vi "Compile.vi"(6 "Python version":string="3.9", 7 "Console":refnum<vi>, 8 "error in":errorcluster, 9 "Code":string="   void setup() {\n    pinMode(LED_BUILTIN, OUTPUT);\n}\n\n   void loop() {\n     digitalWrite(LED_BUILTIN, HIGH);\n     delay(1000);\n     digitalWrite(LED_BUILTIN, LOW);\n     delay(1000);\n}\n", 11 "Arduino in":T1) -> (0 "error out":errorcluster, 1 "standard error":string, 2 "Reply":string, 3 "Arduino out":T1)   [LabVIEW 2022 SP3]
uses:
  ArduinoCtrl.ctl
panel:
  out "resulting string":string
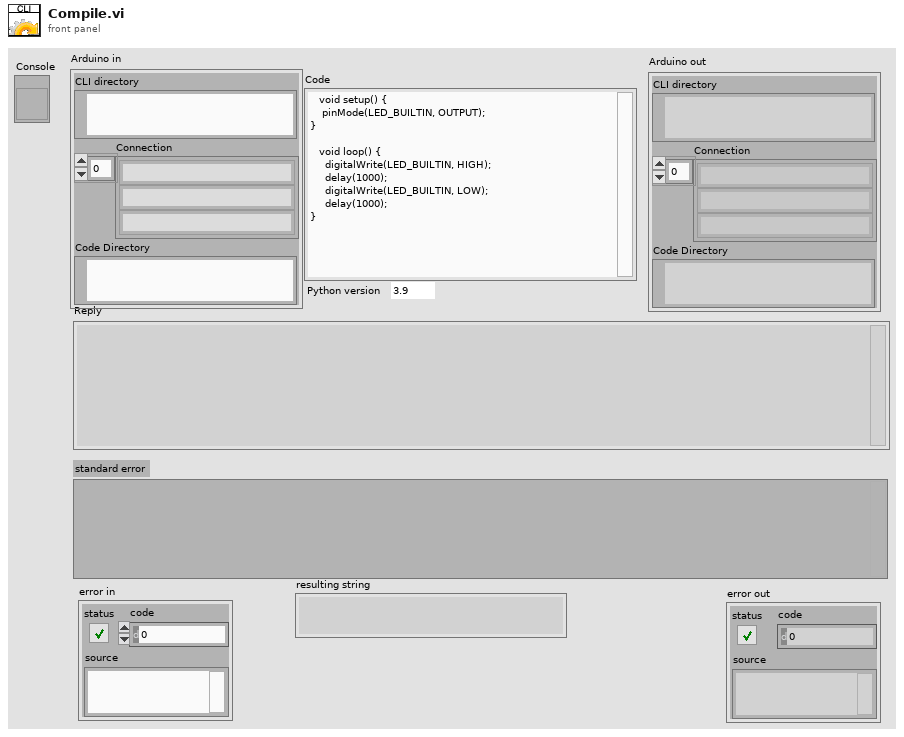
[diagram p1: front panel]
types:
  T1 = typedef "ArduinoCtrl.ctl" = cluster{"CLI directory":path, "Connection":string[], "Code Directory":path}
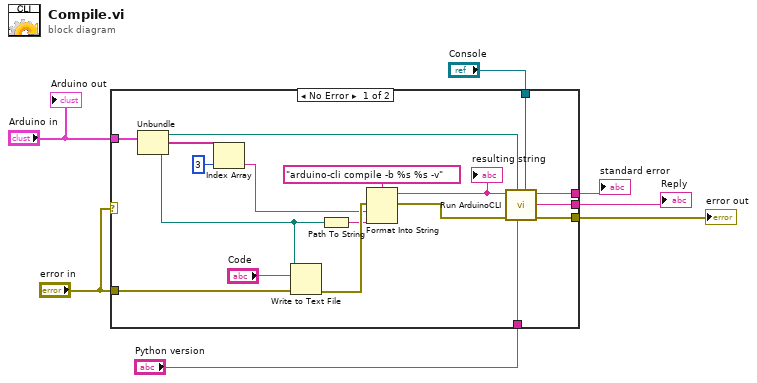
[diagram p0: block diagram]
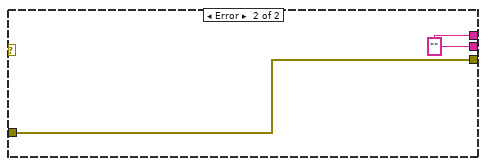
[diagram p2: hidden frame]
diagram:
  n1 = case shown="No Error" "error in" {
    tunnel: [w20 w26] -> w7
    tunnel: "error in" -> [w16 w27]
    tunnel: "Arduino in" -> [w15 _]
    tunnel: [w14 w26] -> w5
    tunnel: [w10 w27] -> w4
    tunnel: "Console" -> [w9 _]
    tunnel: "Python version" -> [w8 _]
    frame No Error {
      n2 = Unbundle(w15) -> ("CLI directory"=w12:path, "Connection"=w19:string[], "Code Directory"=w13:path)
      n3 = Index Array(array=w19, index=3) -> (element=w18:string)
      n4 = Write to Text File(file (use dialog)=w13, text="Code", error in=w16) -> (error out=w22:errorcluster)  [unwired: 1 in, 2 out]
      n5 = Path To String(path=w13) -> (string=w21:string)
      n6 = Format Into String(format string="arduino-cli compile -b %s %s -v" ("command line"), error in=w22, w18, w21) -> (resulting string=w23:string, error out=w11:errorcluster)  [unwired: 1 in]
      "resulting string" <- w23
      n7 = call "Run ArduinoCLI.vi"("Console"=w9, "Python version"=w8, "working directory"=w12, "error in"=w11, "command line"=w23) -> ("error out"=w10:errorcluster, "standard output"=w20:string, "standard error"=w14:string)  [unwired: 4 in]
    }
    frame Error {
      w26 = "" ("standard output")
    }
  }
  "Reply" <- w7
  "standard error" <- w5
  "error out" <- w4
  "Arduino out" <- "Arduino in"
